vi "Check Status No Objects - Synapse CCD.vi"(8 "error in (no error)":errorcluster, 11 "Synapse CCD in":T1={"JYCCDLib.IJYCCDReqd"=refnum, "JYMONOLib.IJYMonoReqd"=refnum, "Integration time"=0.01, "ADC"=0, "GAIN"=0, "areas :"=[[1, 1, 1, 1024, 256, 1, 256]], "Most Recent Data Object"=refnum, "Mono Properties"={"Grating"=0, "Center Wavelength"=0.0, "Entrance Slit"=0.0, "Exit Slit"=0.0}, "Coverage"={"Max"=0.0, "Min"=0.0}, "Multi-Acquisitions"={"Dark Subtract?"=FALSE, "Averaging?"=FALSE, "Cosmic Ray Removal?"=FALSE, "# to Average"=0, "Time Between Acq."=0, "Acquisitions Control Array"=[TRUE], "Raw Data"=[], "Processed Data"=[], "Array of Wavelengths"=[]}, "Channel Names"=["Wavelength", "Signal"], "Channel Units"=["nm", "counts"]} {"ADC" items=["   20 kHz", "1 MHz", "1 MHz Ultra"]; "GAIN" items=["High Light", "Best Dynamic", "High Sensitivity"]; "Mono Properties"."Grating" items=["1200 lines/mm - 500 nm Blaze", "1200 lines/mm - 750 nm Blaze", "600 lines/mm - 1000 nm Blaze"]}) -> (0 "error out":errorcluster, 1 "Status":string, 2 "Ready?":bool, 3 "Synapse CCD out":T1={"JYCCDLib.IJYCCDReqd"=refnum, "JYMONOLib.IJYMonoReqd"=refnum, "Integration time"=0.01, "ADC"=0, "GAIN"=0, "areas :"=[[1, 1, 1, 1024, 256, 1, 256]], "Most Recent Data Object"=refnum, "Mono Properties"={"Grating"=0, "Center Wavelength"=0.0, "Entrance Slit"=0.0, "Exit Slit"=0.0}, "Coverage"={"Max"=0.0, "Min"=0.0}, "Multi-Acquisitions"={"Dark Subtract?"=FALSE, "Averaging?"=FALSE, "Cosmic Ray Removal?"=FALSE, "# to Average"=0, "Time Between Acq."=0, "Acquisitions Control Array"=[TRUE], "Raw Data"=[], "Processed Data"=[], "Array of Wavelengths"=[]}, "Channel Names"=["Wavelength", "Signal"], "Channel Units"=["nm", "counts"]} {"ADC" items=["   20 kHz", "1 MHz", "1 MHz Ultra"]; "GAIN" items=["High Light", "Best Dynamic", "High Sensitivity"]; "Mono Properties"."Grating" items=["1200 lines/mm - 500 nm Blaze", "1200 lines/mm - 750 nm Blaze", "600 lines/mm - 1000 nm Blaze"]})   [LabVIEW 2015]
doc: "(Dynamic) Check if the instrument is powered on and update its member fields with the instrument's current status. Optionally return a text status message."
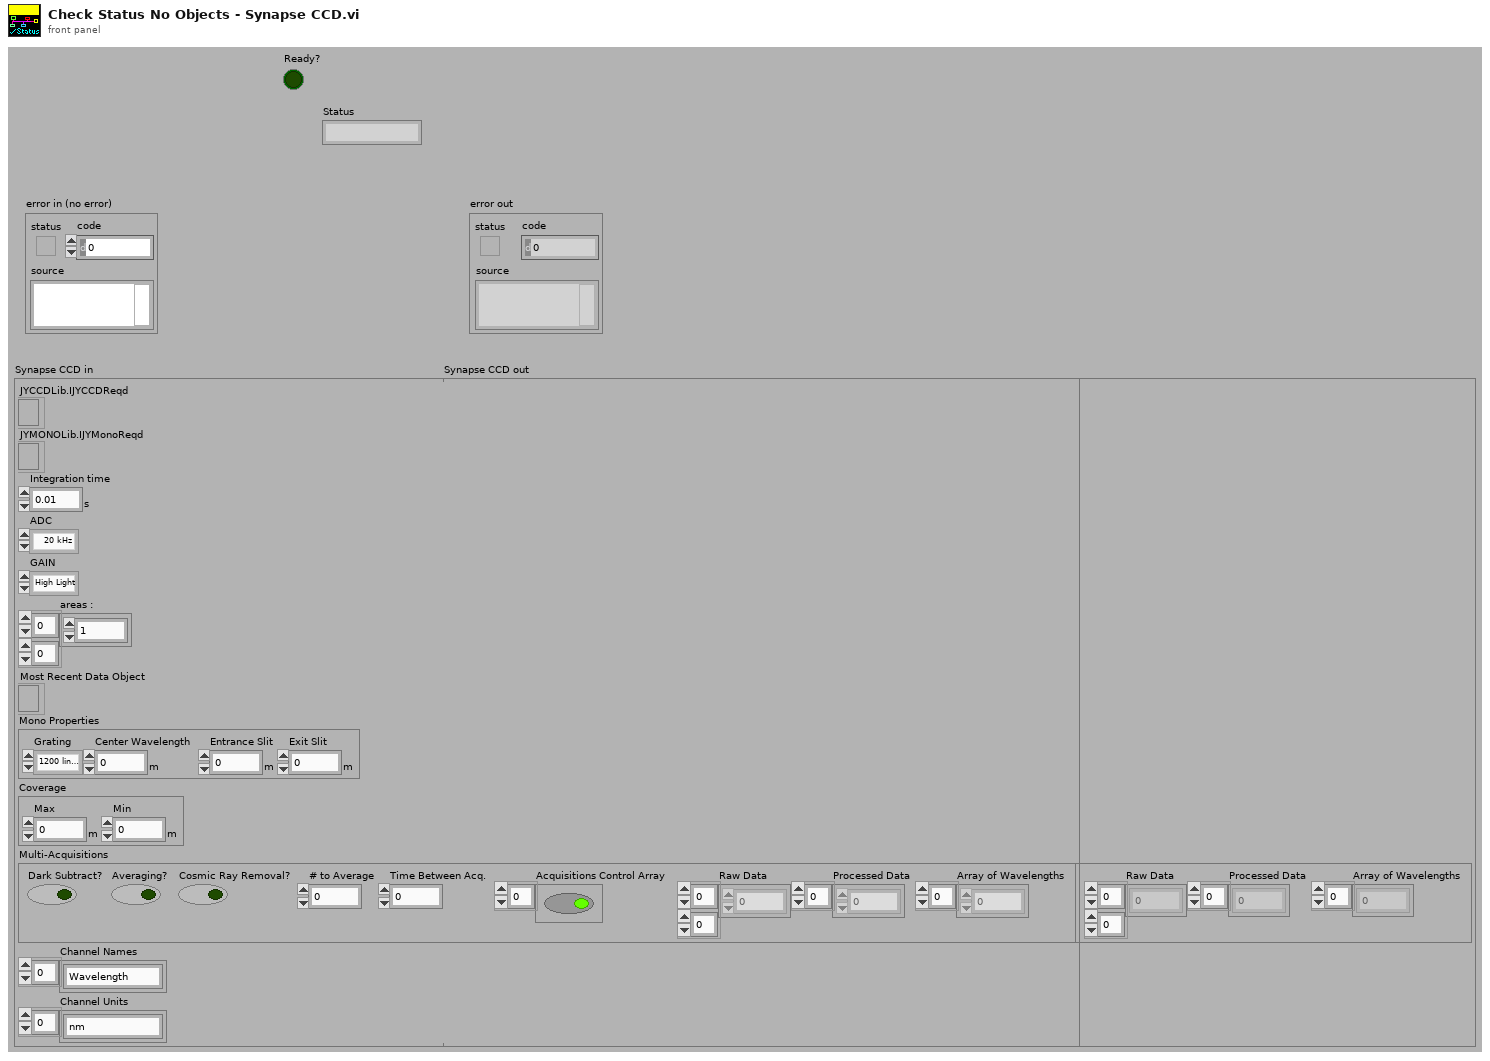
[diagram p1: front panel]
types:
  T1 = cluster{"JYCCDLib.IJYCCDReqd":refnum<k7>, "JYMONOLib.IJYMonoReqd":refnum<k7>, "Integration time":dbl[unit], "ADC":u16, "GAIN":u16, "areas :":i32[][], "Most Recent Data Object":refnum<k7>, "Mono Properties":cluster{"Grating":u16, "Center Wavelength":dbl[unit], "Entrance Slit":dbl[unit], "Exit Slit":dbl[unit]}, "Coverage":cluster{"Max":dbl[unit], "Min":dbl[unit]}, "Multi-Acquisitions":cluster{"Dark Subtract?":bool, "Averaging?":bool, "Cosmic Ray Removal?":bool, "# to Average":u32, "Time Between Acq.":u32, "Acquisitions Control Array":bool[], "Raw Data":i32[][], "Processed Data":dbl[], "Array of Wavelengths":dbl[]}, "Channel Names":string[], "Channel Units":string[]}
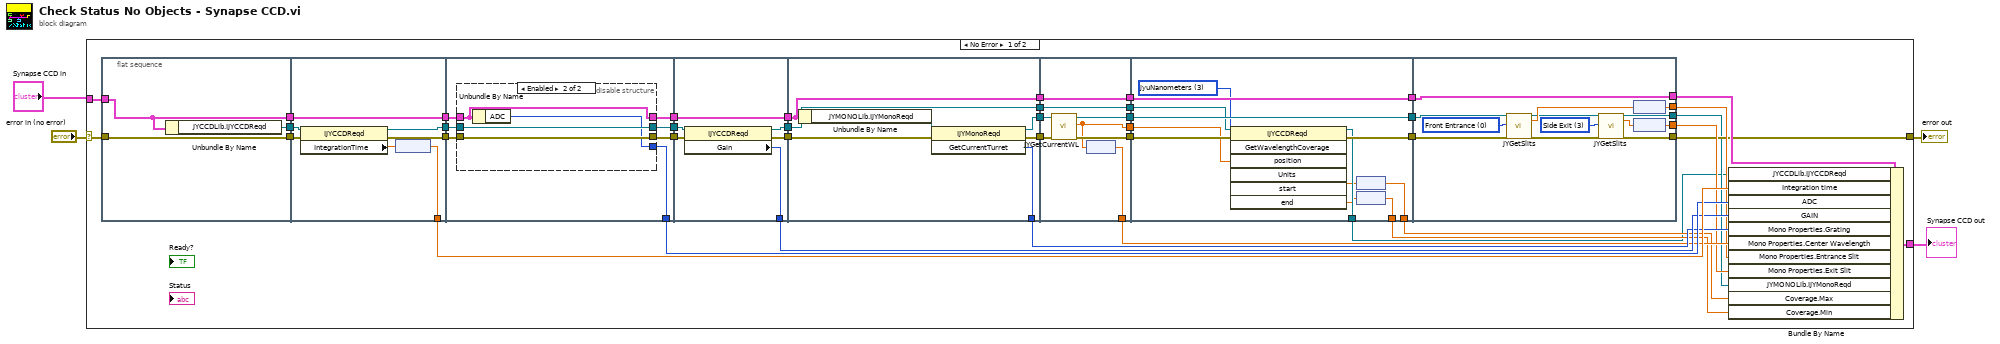
[diagram p0: block diagram]
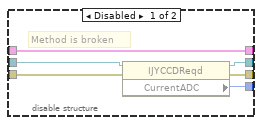
[diagram p2: hidden frame]
diagram:
  n1 = case shown="No Error" "error in (no error)" {
    selector: "error in (no error)" -> [w13 w118]
    tunnel: "Synapse CCD in" -> [w27 w119]
    tunnel: [w25 w119] -> w1
    tunnel: [w17 w118] -> w4
    frame No Error {
      n2 = flat-sequence {
        tunnel: w13 -> [w46]
        tunnel: w27 -> [w45]
        tunnel: [w45] -> w8
        tunnel: [w47] -> w7
        tunnel: [w46] -> w6
        tunnel: [w50] -> w44
        tunnel: w8 -> [w54]
        tunnel: [w54] -> w43
        tunnel: [w51] -> w42
        tunnel: [w52] -> w24
        tunnel: w7 -> [w49]
        tunnel: w6 -> [w48]
        tunnel: w44 -> [w59]
        tunnel: [w58] -> w41
        tunnel: w43 -> [w56]
        tunnel: [w55] -> w40
        tunnel: w42 -> [w61]
        tunnel: [w60] -> w39
        tunnel: [w57] -> w23
        tunnel: w41 -> [w75]
        tunnel: w40 -> [w77]
        tunnel: [w77] -> w12
        tunnel: w39 -> [w76]
        tunnel: [w74] -> w22
        tunnel: [w73] -> w11
        tunnel: [w72] -> w10
        tunnel: w12 -> [w84]
        tunnel: [w81] -> w21
        tunnel: [w84] -> w38
        tunnel: [w82] -> w37
        tunnel: [w80] -> w36
        tunnel: [w78] -> w35
        tunnel: w11 -> [w79]
        tunnel: w10 -> [w78]
        tunnel: w38 -> [w92]
        tunnel: w37 -> [w91]
        tunnel: w36 -> [w89]
        tunnel: [w86] -> w20
        tunnel: [w92] -> w34
        tunnel: [w90] -> w33
        tunnel: [w88] -> w32
        tunnel: w35 -> [w87]
        tunnel: [w87] -> w31
        tunnel: [w85] -> w9
        tunnel: w34 -> [w104]
        tunnel: [w104] -> w30
        tunnel: w33 -> [w102]
        tunnel: w32 -> [w103]
        tunnel: [w103] -> w29
        tunnel: [w101] -> w28
        tunnel: w31 -> [w100]
        tunnel: [w99] -> w5
        tunnel: [w98] -> w15
        tunnel: [w97] -> w14
        tunnel: w9 -> [w96]
        tunnel: [w117] -> w26
        tunnel: w30 -> [w117]
        tunnel: w29 -> [w114]
        tunnel: [w109] -> w19
        tunnel: [w108] -> w18
        tunnel: [w107] -> w17
        tunnel: [w106] -> w16
        tunnel: w28 -> [w105]
        frame #0 {
          n3 = Unbundle By Name(w45) -> ("JYCCDLib.IJYCCDReqd"=w47:refnum<k7>)
        }
        frame #1 {
          n4 = property class="IJYCCDReqd"(reference=w49, error in=w48) -> (reference out=w51:refnum<k7>, error out=w50:errorcluster, "IntegrationTime"=w53:dbl)
          n5 = node(w53) -> (w52:dbl[unit])
        }
        frame #2 {
          n6 = disable-structure shown="Enabled" {
            disable-tunnel: w61 -> [w67 w71]
            disable-tunnel: [w66 w71] -> w60
            disable-tunnel: w59 -> [w65 w70]
            disable-tunnel: [w64 w70] -> w58
            disable-tunnel: [w63 w68] -> w57
            disable-tunnel: w56 -> [w62 w69]
            disable-tunnel: [w62 w69] -> w55
            frame Disabled {
              # "Method is broken"
              n7 = property class="IJYCCDReqd"(reference=w67, error in=w65) -> (reference out=w66:refnum<k7>, error out=w64:errorcluster, "CurrentADC"=w63:i32)
            }
            frame Enabled {
              n8 = Unbundle By Name(w69) -> ("ADC"=w68:u16)
            }
          }
        }
        frame #3 {
          n9 = property class="IJYCCDReqd"(reference=w76, error in=w75) -> (reference out=w72:refnum<k7>, error out=w73:errorcluster, "Gain"=w74:i32)
        }
        frame #4 {
          n10 = Unbundle By Name(w84) -> ("JYMONOLib.IJYMonoReqd"=w83:refnum<k7>)
          n11 = invoke class="IJYMonoReqd" method="GetCurrentTurret"(reference=w83, error in=w79) -> (reference out=w80:refnum<k7>, error out=w82:errorcluster, "GetCurrentTurret"=w81:i32)  [unwired: 1 in]
        }
        frame #5 {
          n12 = call "JYGetCurrentWL.vi"("error in (no error)"=w91, "JYMONOLib.IJYMonoReqd In"=w89) -> ("error out"=w90:errorcluster, "Current WL"=w85:dbl, "JYMONOLib.IJYMonoReqd Out"=w88:refnum<k7>)  [unwired: 6 in, 1 out]
          n13 = node(w85) -> (w86:dbl[unit])
        }
        frame #6 {
          w95 = 3 items=["jyuUndefined", "jyuMillimeters", "jyuMicrons", "jyuNanometers", "jyuAngstroms", "jyuPicometers", "jyuBandpass", "jyuSteps", "jyuWavenumbers", "jyuDeltaWavenumbers", "jyuElectronVolts", "jyuNanoseconds", "jyuMicroseconds", "jyuMilliseconds", "jyuSeconds", "jyuMinutes", "jyuHours", "jyuVolts", "jyuMillivolts", "jyuMicrovolts", "jyuAmperes", "jyuMilliAmps", "jyuMicroAmps", "jyuCounts", "jyuCountsPerSecond", "jyuDegreesCelcius", "jyuDegreesFahrenheit", "jyuDegreesKelvin", "jyuPixels", "jyuTotalUnitsPlusOne"] ("Units")
          n14 = invoke class="IJYCCDReqd" method="GetWavelengthCoverage"(reference=w100, error in=w102, "position"=w96, "Units"=w95) -> (reference out=w99:refnum<k7>, error out=w101:errorcluster, "start"=w94:dbl, "end"=w93:dbl)  [unwired: 3 in, 3 out]
          n15 = node(w94) -> (w98:dbl[unit])
          n16 = node(w93) -> (w97:dbl[unit])
        }
        frame #7 {
          w115 = u16 0 items=["Front Entrance", "Side Entrance", "Front Exit", "Side Exit", "First Intermediate", "Second Intermediate"] ("Slit")
          w116 = u16 3 items=["Front Entrance", "Side Entrance", "Front Exit", "Side Exit", "First Intermediate", "Second Intermediate"] ("Slit")
          n17 = call "JYGetSlits.vi"("MonoRefNum IN"=w114, "Slit"=w115, "error in (no error)"=w105) -> ("MonoRefNum Out"=w111:refnum<k7>, "Slit Width"=w113:dbl, "error out"=w112:errorcluster)  [unwired: 13 in, 1 out]
          n18 = call "JYGetSlits.vi"("MonoRefNum IN"=w111, "Slit"=w116, "error in (no error)"=w112) -> ("MonoRefNum Out"=w106:refnum<k7>, "Slit Width"=w110:dbl, "error out"=w107:errorcluster)  [unwired: 13 in, 1 out]
          n19 = node(w113) -> (w109:dbl[unit])
          n20 = node(w110) -> (w108:dbl[unit])
        }
      }
      n21 = Bundle By Name(cluster=w26, "JYCCDLib.IJYCCDReqd"=w5, "Integration time"=w24, "ADC"=w23, "GAIN"=w22, "Mono Properties.Grating"=w21, "Mono Properties.Center Wavelength"=w20, "Mono Properties.Entrance Slit"=w19, "Mono Properties.Exit Slit"=w18, "JYMONOLib.IJYMonoReqd"=w16, "Coverage.Max"=w15, "Coverage.Min"=w14) -> (w25:T1)
    }
    frame Error {
    }
  }
  "error out" <- w4
  "Synapse CCD out" <- w1
